vi "SR830_Test.vi"() -> ()   [LabVIEW 2020]
panel:
  in  "退出":bool
  in  "数据长度":dbl
  in  "Sample Rate (0: 62.5 mHz)":u16(ring)=11 items=["62.5 mHz", "125 mHz", "250 mHz", "500 mHz", "1 Hz", "2 Hz", "4 Hz", "8Hz", "16 Hz", "32 Hz", "64 Hz", "128 Hz", "256 Hz", "512 Hz", "Trigger "]
  in  "VISA 输入":refnum<visa-resource-name>="GPIB0::7::INSTR"
  out "Channel 2":sgl[](graph)
  out "Channel 1":sgl[](graph)
  out "Channel 2 数值":dbl format="%#_6f"
  out "Channel 1 数值":dbl format="%#_6f"
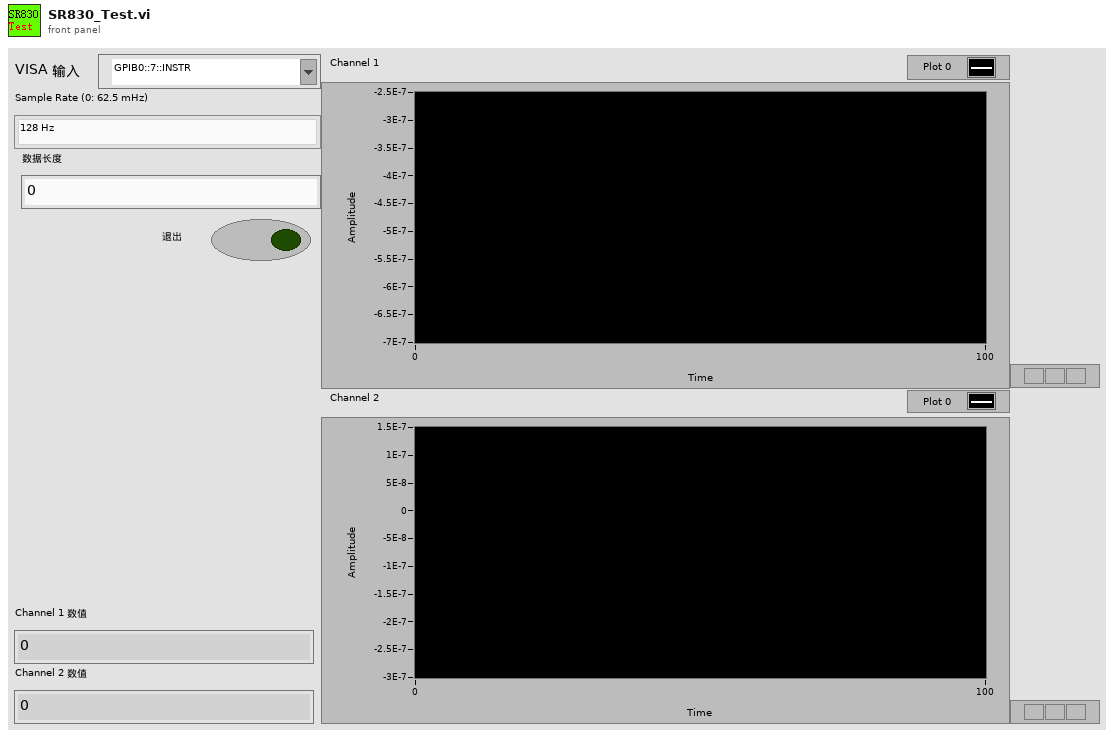
[diagram p1: front panel]
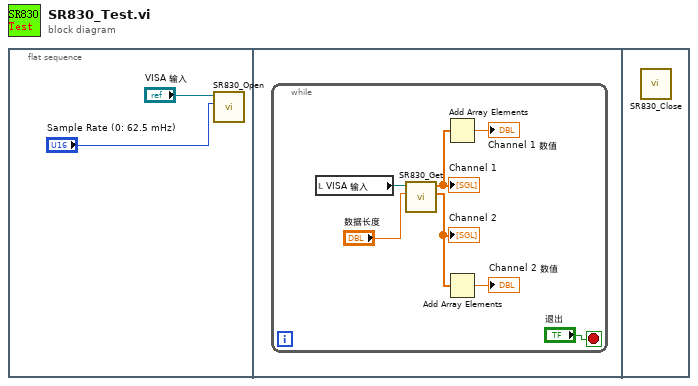
[diagram p0: block diagram]
diagram:
  n1 = flat-sequence {
    frame #0 {
      n2 = call "SR830_Open.vi"("Sample Rate (0: 62.5 mHz)"="Sample Rate (0: 62.5 mHz)", "VISA 输入"="VISA 输入") -> ()  [unwired: 9 in, 1 out]
    }
    frame #1 {
      n3 = while {
        stop <- "退出" stop-if-true
        n4 = local read "VISA 输入"() -> (w7:refnum<visa-resource-name>)
        n5 = call "SR830_Get.vi"("数据长度"="数据长度", "VISA 输入"=w7) -> ("Channel 2"=w4:sgl[], "Channel 1"=w6:sgl[])  [unwired: 7 in, 1 out]
        "Channel 1" <- w6
        "Channel 2" <- w4
        n6 = Add Array Elements(numeric array=w6) -> (sum=→"Channel 1 数值":sgl)
        n7 = Add Array Elements(numeric array=w4) -> (sum=→"Channel 2 数值":sgl)
      }
    }
    frame #2 {
      n8 = call "SR830_Close.vi"() -> ()  [unwired: 11 in, 1 out]
    }
  }
